vi "determineTargetType.vi"(8 "error in (no error)":errorcluster, 10 "childAttributes":T1[](array[typedef])) -> (0 "error out":errorcluster, 3 "Difftrack.lvclass":refnum<class "Difftrack.lvclass">)   [LabVIEW 2022 SP3, in "TCSDataDefinitions.lvlib" / "TCSCommand.lvlib" / "TargetConfiguration.lvlib" / "Target.lvlib" / "Difftrack.lvclass"]
uses:
  Difftrack.lvclass
  <userlib>/Common/XML/Typedefs/AttributeElements.ctl
  DifftrackAzEl/DifftrackAzEl.lvclass
  C:/Development/rimas/RIMAS/TCS/TCS_external_interfaces/TCSDataDefinitions/TCSCommand/TargetConfiguration/Target/Difftrack/Difftrack.lvclass
  DifftrackRADec/DifftrackRADec.lvclass
  <userlib>/Common/XML/XML.lvlib
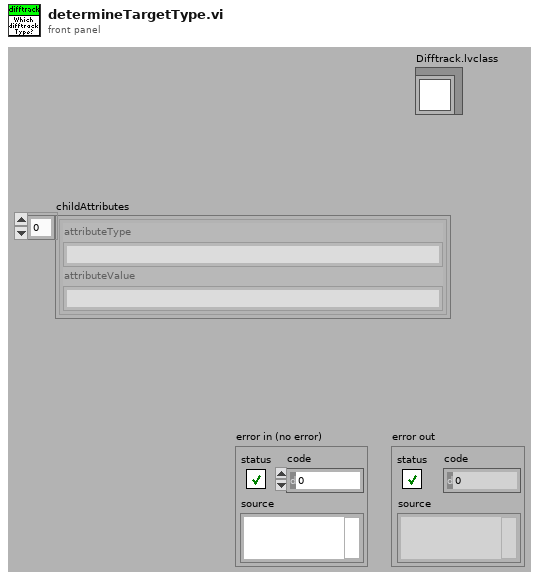
[diagram p1: front panel]
types:
  T1 = typedef "XML.lvlib/AttributeElements.ctl" = cluster{"attributeType":string, "attributeValue":string}
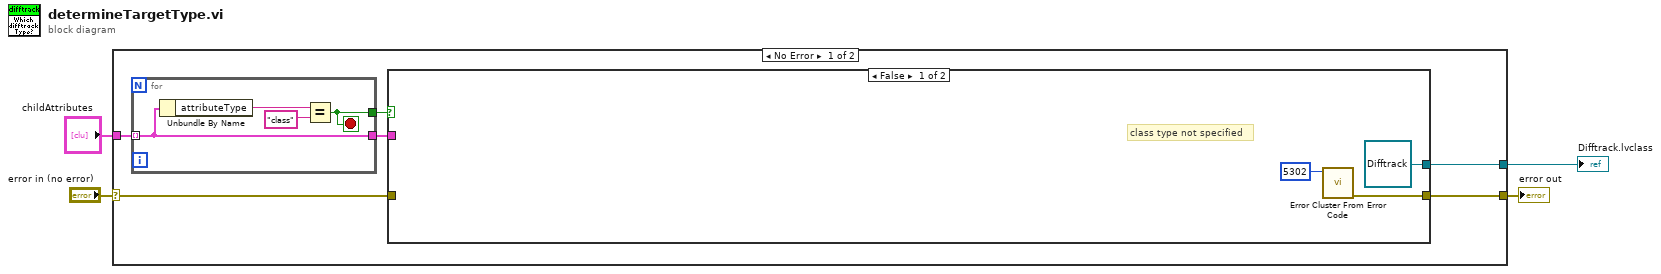
[diagram p0: block diagram]
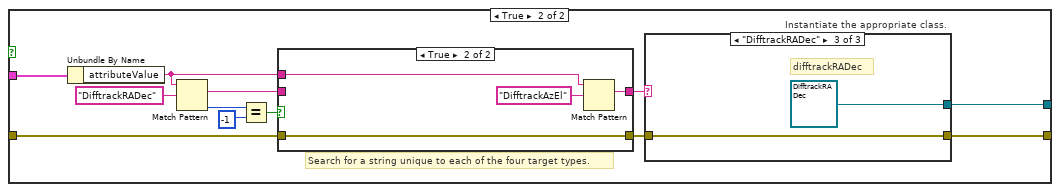
[diagram p2: hidden frame]
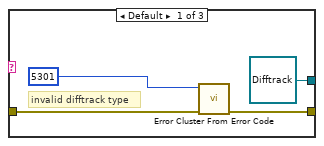
[diagram p3: hidden frame]
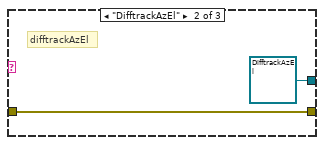
[diagram p4: hidden frame]
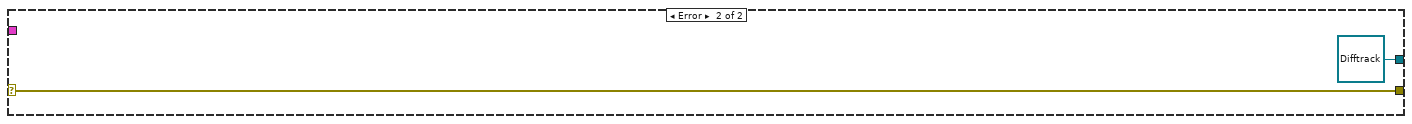
[diagram p6: hidden frame]
diagram:
  n1 = case shown="No Error" "error in (no error)" {
    selector: "error in (no error)" -> [w10 w44]
    tunnel: [w6 w44] -> w3
    tunnel: [w9 refnum<class "Difftrack.lvclass"> refnum ("Difftrack.lvclass")] -> w2
    tunnel: "childAttributes" -> [w7 _]
    frame No Error {
      n2 = for {
        tunnel: w7 -> [w12] mode=indexing
        tunnel: [w12] -> w8
        tunnel: [w11] -> w5
        stop <- w11 stop-if-true
        n3 = Unbundle By Name(w12) -> ("attributeType"=w13:string)
        n4 = Equal?(x=w13, y="class") -> (x = y?=w11:bool)
      }
      n5 = case shown="False" w5 {
        tunnel: w8 -> [_ w29]
        tunnel: w10 -> [_ w28]
        tunnel: [refnum<class "Difftrack.lvclass"> refnum ("Difftrack.lvclass") w27] -> w9
        tunnel: [w16 w26] -> w6
        frame False {
          # "class type not specified"
          n6 = call <vilib>:"Error Cluster From Error Code.vi"("error code (0)"=5302 ("code")) -> ("error out"=w16:errorcluster)  [unwired: 8 in]
        }
        frame True {
          # "Search for a string unique to each of the four target types."
          n7 = Unbundle By Name(w29) -> ("attributeValue"=w25:string)
          n8 = Match Pattern(string=w25, regular expression="DifftrackRADec") -> (match substring=w20:string, offset past match=w23:i32)  [unwired: 1 in, 2 out]
          n9 = Equal?(x=w23, y=-1) -> (x = y?=w21:bool)
          n10 = case shown="True" w21 {
            tunnel: w25 -> [_ w41]
            tunnel: w28 -> [_ w40]
            tunnel: [_ w40] -> w18
            tunnel: [w38 w39] -> w19
            tunnel: w20 -> [w38 _]
            frame False {
            }
            frame True {
              n11 = Match Pattern(string=w41, regular expression="DifftrackAzEl") -> (match substring=w39:string)  [unwired: 1 in, 3 out]
            }
          }
          n12 = case "Instantiate the appropriate class." shown="\"DifftrackRADec\"" w19 {
            tunnel: w18 -> [w31 w35 w37]
            tunnel: [w30 w35 w37] -> w26
            tunnel: [refnum<class "Difftrack.lvclass"> refnum ("Difftrack.lvclass") refnum<class "DifftrackAzEl.lvclass"> refnum ("DifftrackAzEl.lvclass") refnum<class "DifftrackRADec.lvclass"> refnum ("DifftrackRADec.lvclass")] -> w27
            frame Default {
              # "invalid difftrack type"
              n13 = call <vilib>:"Error Cluster From Error Code.vi"("error in (no error)"=w31, "error code (0)"=5301 ("code")) -> ("error out"=w30:errorcluster)  [unwired: 7 in]
            }
            frame "DifftrackAzEl" {
              # "difftrackAzEl"
            }
            frame "DifftrackRADec" {
              # "difftrackRADec"
            }
          }
        }
      }
    }
    frame Error {
    }
  }
  "error out" <- w3
  "Difftrack.lvclass" <- w2
